vi "Test.vi"   [LabVIEW 2020]
doc: "This VI is called when test mode begins, and will automatically be terminated when it ends. You can add manual or automatic tests and invoke them from the dashboard."
uses:
  <vilib>/Rock Robotics/WPI/ThirdParty/REV Robotics/REVLib/Typedef/Spark MAX Control Type.ctl
types:
  T1 = typedef "WPI_MotorControlDeviceRef.ctl" = cluster{"DeviceStatus":errorcluster, "Type":T2, "PWM":cluster{"PWM Channel":T3, "DeadBand":T4}, "CAN":cluster{"Device Number":u8, "SetOutput VI Ref":variant, "GetOutput VI Ref":variant, "Enable VI Ref":variant, "Disable VI Ref":variant, "Data":variant}, "Invert":bool, "DIO PWM":cluster{"PWM \"Enable\" Channel":T3, "DIOChannel":T5, "PWM Rate":dbl}}
  T2 = typedef "WPI_MotorControlType.ctl" = enum16{"PWM", "CAN", "DIO PWM"}
  T3 = typedef "FPGA_DIOPWMChannel.ctl" = enum8{"PWM 0", "PWM 1", "PWM 2", "PWM 3", "PWM 4", "PWM 5", "PWM 6", "PWM 7", "PWM 8", "PWM 9", "PWM MXP 0", "PWM MXP 1", "PWM MXP 2", "PWM MXP 3", "PWM MXP 4", "PWM MXP 5", "PWM MXP 6", "PWM MXP 7", "PWM MXP 8", "PWM MXP 9", "Invalid"}
  T4 = typedef "WPI_PWMDeadband.ctl" = cluster{"Name":string, "maxPositivePwm":i32, "minPositivePwm":i32, "centerPwm":i32, "maxNegativePwm":i32, "minNegativePwm":i32, "angularRange":u16}
  T5 = typedef "FPGA_DIOChannel.ctl" = enum8{"DIO 0", "DIO 1", "DIO 2", "DIO 3", "DIO 4", "DIO 5", "DIO 6", "DIO 7", "DIO 8", "DIO 9", "DIO MXP 0", "DIO MXP 1", "DIO MXP 2", "DIO MXP 3", "DIO MXP 4", "DIO MXP 5", "DIO MXP 6", "DIO MXP 7", "DIO MXP 8", "DIO MXP 9", "DIO MXP 10", "DIO MXP 11", "DIO MXP 12", "DIO MXP 13", "DIO MXP 14", "DIO MXP 15", "SPI Port CS1", "SPI Port CS2", "SPI Port CS3", "SPI Port MISO", "SPI Port MOSI", "Invalid"}
  T6 = typedef "Spark MAX Control Type.ctl" = enum16{"Percent VBus", "Voltage", "Velocity", "Position", "Smart Motion", "Current", "Smart Velocity"}
  T7 = typedef "Joystick_Controls.ctl" = cluster{"Pilot Left Joystick X":dbl, "Pilot Left Joystick Y":dbl, "Pilot X Button":bool, "Pilot Circle Button":bool, "Pilot Square Button":bool, "Pilot Triangle Button":bool, "Pilot Left Bumper":bool, "Pilot Right Bumper":bool, "Pilot Share Button":bool, "Pilot Options Button":bool, "Pilot Left Joystick Press":bool, "Pilot Right Joystick Press":bool, "Pilot Left Trigger":dbl, "Pilot Right Joystick X":dbl, "Pilot Right Joystick Y":dbl, "Pilot Right Trigger":dbl, "Copilot Left Joystick X":dbl, "Copilot Left Joystick Y":dbl, "Copilot X Button":bool, "Copilot Circle Button":bool, "Copilot Square Button":bool, "Copilot Triangle Button":bool, "Copilot Left Bumper":bool, "Copilot Right Bumper":bool, "Copilot Share Button":bool, "Copilot Options Button":bool, "Copilot Left Joystick Press":bool, "Copilot Right Joystick Press":bool, "Copilot Left Trigger":dbl, "Copilot Right Joystick X":dbl, "Copilot Right Joystick Y":dbl, "Copilot Right Trigger":dbl, "Pilot D-pad North":bool, "Pilot D-pad South":bool, "Pilot D-pad East":bool, "Pilot D-pad West":bool, "Pilot D-pad NE ":bool, "Pilot D-pad SE":bool, "Pilot D-pad SW":bool, "Pilot D-pad NW":bool, "CoPilot D-pad North":bool, "CoPilot D-pad South":bool, "CoPilot D-pad East":bool, "CoPilot D-pad West":bool, "CoPilot D-pad NE":bool, "CoPilot D-pad SE":bool, "CoPilot D-pad SW":bool, "CoPilot D-pad NW":bool, "Pilot Left Trigger Pressed":bool, "Pilot Right Trigger Pressed":bool, "CoPilot Left Trigger Pressed":bool, "CoPilot Right Trigger Pressed":bool, "Pilot Left Trigger Firmly":bool, "Pilot Right Trigger Firmly":bool, "Pilot Touchpad":bool, "Pilot PS Button":bool, "CoPilot Left Trigger Firmly":bool, "CoPilot Right Trigger Firmly":bool, "CoPilot Touchpad":bool, "CoPilot PS Button":bool}
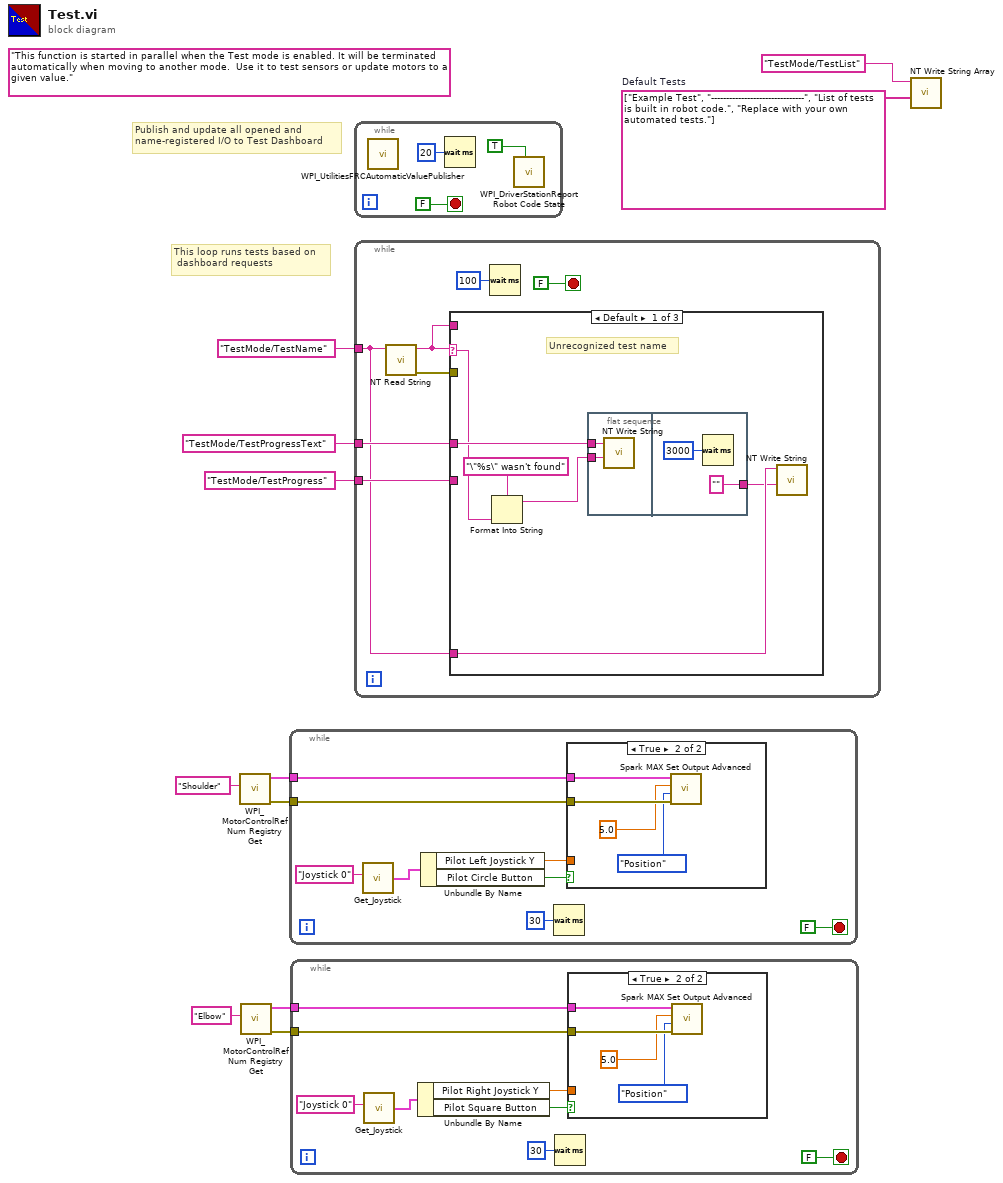
[diagram p0: block diagram]
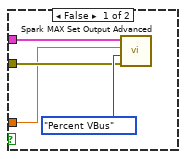
[diagram p2: hidden frame]
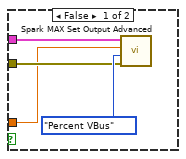
[diagram p3: hidden frame]
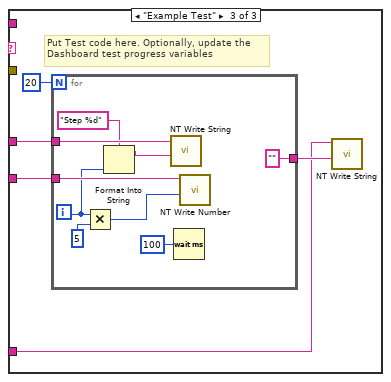
[diagram p5: hidden frame]
diagram:
  w8 = string[] ["Example Test", "-------------------------------", "List of tests is built in robot code.", "Replace with your own automated tests."]  # Default Tests
  (unwired) "This function is started in parallel when the Test mode is enabled. It will be terminated automatically when moving to another mode.  Use it to test sensors or update motors to a given value."
  # "This loop runs tests based on \n dashboard requests"
  # "Publish and update all opened and\nname-registered I/O to Test Dashboard"
  n1 = call <vilib>:"WPI_MotorControlRefNum Registry Get.vi"("refnum name"="Shoulder") -> ("error out"=w4:errorcluster, "MotorControlDevRef"=w5:T1)  [unwired: 9 in]
  n2 = call <vilib>:"WPI_MotorControlRefNum Registry Get.vi"("refnum name"="Elbow") -> ("error out"=w1:errorcluster, "MotorControlDevRef"=w2:T1)  [unwired: 9 in]
  n3 = while {
    tunnel: w5 -> [w16]
    tunnel: w4 -> [w15]
    stop <- FALSE stop-if-true
    n4 = call "Get_Joystick.vi"("Joystick_One"="Joystick 0") -> ("Joystick_Out"=w18:T7)  [unwired: 6 in]
    n5 = Unbundle By Name(w18) -> ("Pilot Left Joystick Y"=w14:dbl, "Pilot Circle Button"=w17:bool)
    n6 = Wait (ms)(milliseconds to wait=u32 30) -> ()  [unwired: 1 out]
    n7 = case shown="True" w17 {
      tunnel: w16 -> [w21 w27]
      tunnel: w15 -> [w22 w26]
      tunnel: w14 -> [w20 _]
      frame False {
        n8 = call <vilib>:"Spark MAX Set Output Advanced.vi"("error in (no error)"=w22, "Control Mode"=Spark_MAX_Control_Type."Percent VBus", "Setpoint"=w20, "MotorControlDevRef"=w21) -> ()  [unwired: 6 in, 2 out]
      }
      frame True {
        n9 = call <vilib>:"Spark MAX Set Output Advanced.vi"("error in (no error)"=w26, "Control Mode"=Spark_MAX_Control_Type."Position", "Setpoint"=5.0, "MotorControlDevRef"=w27) -> ()  [unwired: 6 in, 2 out]
      }
    }
  }
  n10 = while {
    tunnel: w2 -> [w32]
    tunnel: w1 -> [w31]
    stop <- FALSE stop-if-true
    n11 = call "Get_Joystick.vi"("Joystick_One"="Joystick 0") -> ("Joystick_Out"=w34:T7)  [unwired: 6 in]
    n12 = Unbundle By Name(w34) -> ("Pilot Right Joystick Y"=w30:dbl, "Pilot Square Button"=w33:bool)
    n13 = Wait (ms)(milliseconds to wait=u32 30) -> ()  [unwired: 1 out]
    n14 = case shown="True" w33 {
      tunnel: w32 -> [w37 w43]
      tunnel: w31 -> [w38 w42]
      tunnel: w30 -> [w36 _]
      frame False {
        n15 = call <vilib>:"Spark MAX Set Output Advanced.vi"("error in (no error)"=w38, "Control Mode"=Spark_MAX_Control_Type."Percent VBus", "Setpoint"=w36, "MotorControlDevRef"=w37) -> ()  [unwired: 6 in, 2 out]
      }
      frame True {
        n16 = call <vilib>:"Spark MAX Set Output Advanced.vi"("error in (no error)"=w42, "Control Mode"=Spark_MAX_Control_Type."Position", "Setpoint"=5.0, "MotorControlDevRef"=w43) -> ()  [unwired: 6 in, 2 out]
      }
    }
  }
  n17 = while {
    stop <- FALSE stop-if-true
    n18 = call <vilib>:"WPI_UtilitiesFRCAutomaticValuePublisher.vi"() -> ()  [unwired: 12 in]
    n19 = Wait (ms)(milliseconds to wait=u32 20) -> ()  [unwired: 1 out]
    n20 = call <vilib>:"WPI_DriverStationReport Robot Code State.vi"("Test"=TRUE ("Autonomous")) -> ()  [unwired: 10 in, 1 out]
  }
  n21 = while {
    tunnel: "TestMode/TestName" ("Name") -> [w48]
    tunnel: "TestMode/TestProgressText" ("Name") -> [w51]
    tunnel: "TestMode/TestProgress" ("Name") -> [w50]
    stop <- FALSE stop-if-true
    n22 = call <vilib>:"NT Read String.vi"("name"=w48) -> ("error out"=w47:errorcluster, "value"=w49:string)  [unwired: 8 in, 1 out]
    n23 = case shown="Default" w49 {
      selector: w49 -> [w58 _ _]
      tunnel: w48 -> [w55 _ w64]
      tunnel: w51 -> [w59 _ w67]
      tunnel: w50 -> [_ _ w68]
      tunnel: w49 -> [_ _ _]
      tunnel: w47 -> [_ _ _]
      frame Default {
        # "Unrecognized test name"
        n24 = Format Into String(format string="\"%s\" wasn't found" ("Name"), w58) -> (resulting string=w57:string)  [unwired: 2 in, 1 out]
        n25 = flat-sequence {
          tunnel: w59 -> [w60]
          tunnel: w57 -> [w61]
          tunnel: ["" ("Name")] -> w54
          frame #0 {
            n26 = call <vilib>:"NT Write String.vi"("value"=w61, "name"=w60) -> ()  [unwired: 9 in, 1 out]
          }
          frame #1 {
            n27 = Wait (ms)(milliseconds to wait=u32 3000) -> ()  [unwired: 1 out]
          }
        }
        n28 = call <vilib>:"NT Write String.vi"("value"=w54, "name"=w55) -> ()  [unwired: 9 in, 1 out]
      }
      frame "" {
        # "No test to run"
      }
      frame "Example Test" {
        # "Put Test code here. Optionally, update the\nDashboard test progress variables"
        n29 = for {
          N: 20 -> [_]
          tunnel: w68 -> [w77]
          tunnel: w67 -> [w75]
          tunnel: ["" ("String")] -> w65
          i -> [w72]
          n30 = Multiply(x=w72, y=u32 5 ("milliseconds to wait")) -> (x*y=w73:u32)
          n31 = Format Into String(format string="Step %d", w72) -> (resulting string=w70:string)  [unwired: 2 in, 1 out]
          n32 = call <vilib>:"NT Write String.vi"("value"=w70, "name"=w75) -> ()  [unwired: 9 in, 1 out]
          n33 = Wait (ms)(milliseconds to wait=u32 100) -> ()  [unwired: 1 out]
          n34 = call <vilib>:"NT Write Number.vi"("value"=w73, "name"=w77) -> ()  [unwired: 9 in, 1 out]
        }
        n35 = call <vilib>:"NT Write String.vi"("value"=w65, "name"=w64) -> ()  [unwired: 9 in, 1 out]
      }
    }
    n36 = Wait (ms)(milliseconds to wait=u32 100) -> ()  [unwired: 1 out]
  }
  n37 = call <vilib>:"NT Write String Array.vi"("value"=w8, "name"="TestMode/TestList" ("Name")) -> ()  [unwired: 9 in, 1 out]
